vi "FA_ConvertToConfigItemData.vi"(8 "Error In":errorcluster, 11 "XML String":string) -> (0 "Error Out":errorcluster, 3 "Items":T1)   [LabVIEW 2014, in "FA_NativeTypes.lvlib"]
doc: "Converts from an XML string to the items typedef"
uses:
  FA_NativeTypes.lvlib
  FA_ConfigItem.ctl
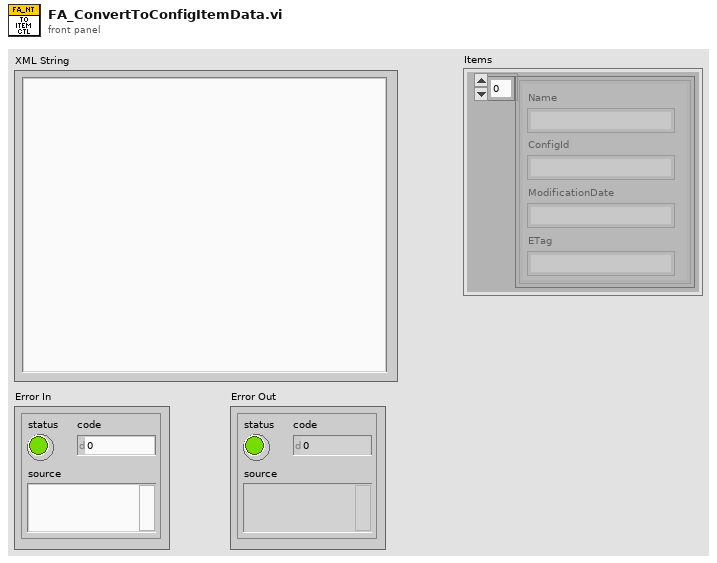
[diagram p1: front panel]
types:
  T1 = typedef "FA_NativeTypes.lvlib/FA_ConfigItem.ctl" = cluster{"Item":cluster{"Name":string, "ConfigId":string, "ModificationDate":string, "ETag":string}[]}
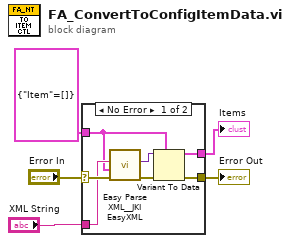
[diagram p0: block diagram]
diagram:
  n1 = case shown="No Error" "Error In" {
    selector: "Error In" -> [w12 w14]
    tunnel: [w8 w14] -> w4
    tunnel: [w9 w13] -> w1
    tunnel: "XML String" -> [w7 _]
    tunnel: T1 {"Item"=[]} ("Items") -> [w6 w13]
    frame No Error {
      n2 = call <vilib>:"Easy Parse XML__JKI EasyXML.vi"("error in (no error)"=w12, "LabVIEW Data (Type)"=w6, "XML String"=w7) -> ("error out"=w11:errorcluster, "LabVIEW Data"=w10:variant)  [unwired: 7 in]
      n3 = Variant To Data(error in=w11, type=w6, Variant=w10) -> (data=w9:T1, error out=w8:errorcluster)
    }
    frame Error {
    }
  }
  "Error Out" <- w4
  "Items" <- w1
